vi "AlliGator Find FLI Dataset Paths.vi"(8 "error in (no error)":errorcluster, 11 "Path in":path) -> (0 "error out":errorcluster, 3 "Dataset Paths Array":path[](array[path]))   [LabVIEW 2021, in "AlliGator Files.lvlib"]
doc: "Analyze what type of files or folders the path contains."
uses:
  AlliGator Files.lvlib
  53ac5bec-de5c-4618-965b-4e0dad36e136.vi
  <vilib>/Utility/error.llb/Error Cluster From Error Code.vi
  <vilib>/ErrorRing/Error Ring.xnode
  <userlib>/_OpenG.lib/file/file.llb/openg_file.lvlib
panel:
  out "# Images":i32
  out "# Datasets":i32
  out "Gate Image Folder?":bool
  # "see the AlliGator License on the block diagram (Ctrl+E or Window:Show Block Diagram)"
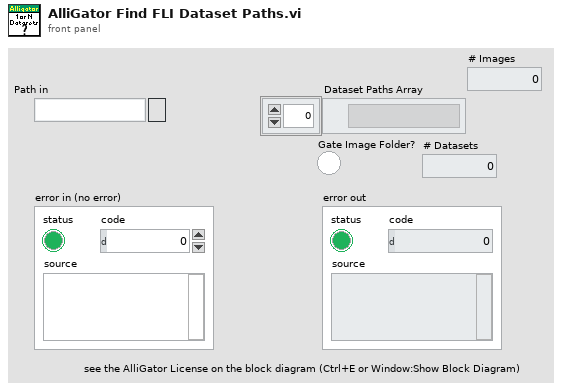
[diagram p1: front panel]
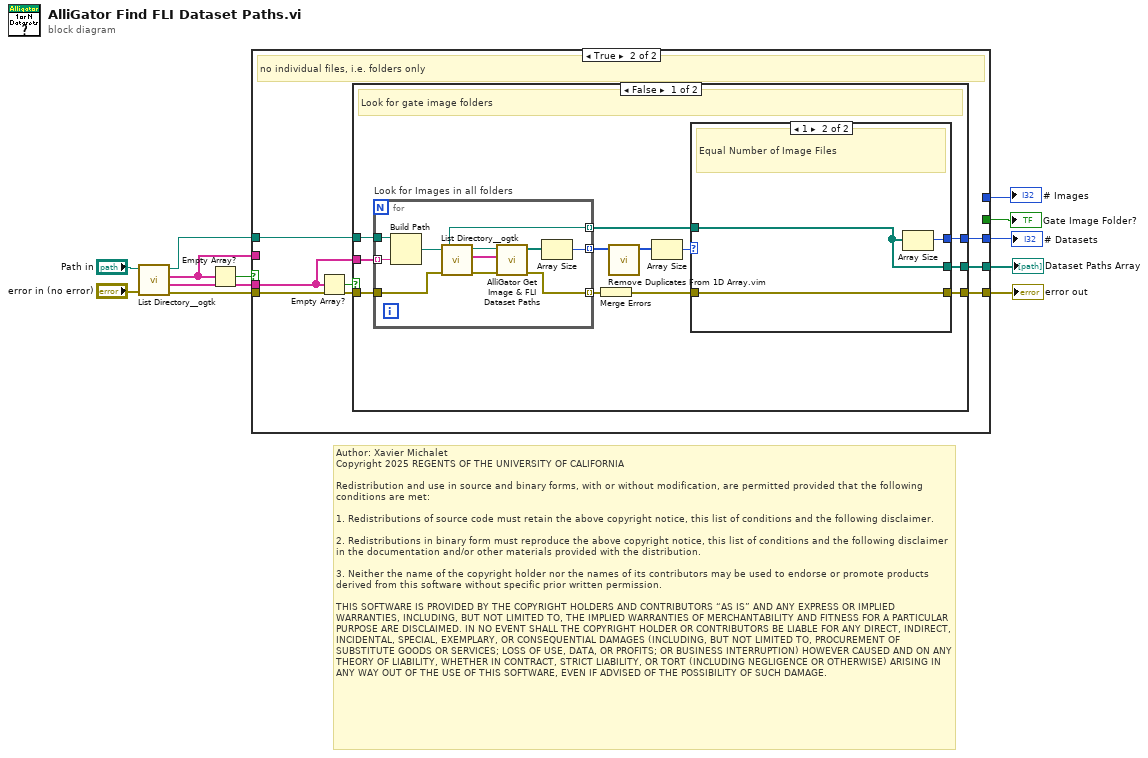
[diagram p0: block diagram]
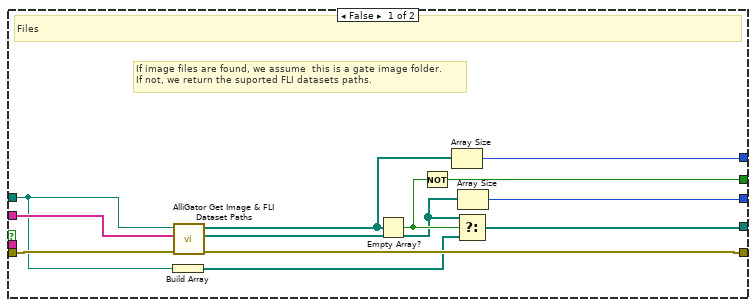
[diagram p2: hidden frame]
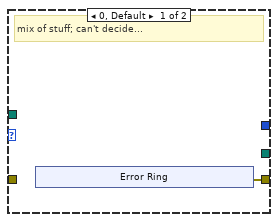
[diagram p3: hidden frame]
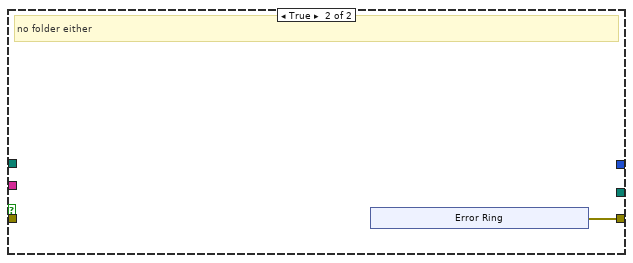
[diagram p4: hidden frame]
diagram:
  # "Author: Xavier Michalet\nCopyright 2025 REGENTS OF THE UNIVERSITY OF CALIFORNIA\n\nRedistribution and use in source and binary forms, with or without modification, are permitted provided that the following conditions are met:\n\n1. Redistributions of source code must retain the above copyright notice, this list of conditions and the following disclaimer.\n\n2. Redistributions in binary form must reproduce the above copyright notice, this list of conditions and the following disclaimer in the documentation and/or other materials provided with the distribution.\n\n3. Neither the name of the copyright holder nor the names of its contributors may be used to endorse or promote products derived from this software without specific prior written permission.\n\nTHIS SOFTWARE IS PROVIDED BY THE COPYRIGHT HOLDERS AND CONTRIBUTORS “AS IS” AND ANY EXPRESS OR IMPLIED WARRANTIES, INCLUDING, BUT NOT LIMITED TO, THE IMPLIED WARRANTIES OF MERCHANTABILITY AND FITNESS FOR A PARTICULAR PURPOSE ARE DISCLAIMED. IN NO EVENT SHALL THE COPYRIGHT HOLDER OR CONTRIBUTORS BE LIABLE FOR ANY DIRECT, INDIRECT, INCIDENTAL, SPECIAL, EXEMPLARY, OR CONSEQUENTIAL DAMAGES (INCLUDING, BUT NOT LIMITED TO, PROCUREMENT OF SUBSTITUTE GOODS OR SERVICES; LOSS OF USE, DATA, OR PROFITS; OR BUSINESS INTERRUPTION) HOWEVER CAUSED AND ON ANY THEORY OF LIABILITY, WHETHER IN CONTRACT, STRICT LIABILITY, OR TORT (INCLUDING NEGLIGENCE OR OTHERWISE) ARISING IN ANY WAY OUT OF THE USE OF THIS SOFTWARE, EVEN IF ADVISED OF THE POSSIBILITY OF SUCH DAMAGE."
  n1 = call <userlib>:"List Directory__ogtk.vi"("error in (no error)"="error in (no error)", "directory path"="Path in") -> ("error out"=w6:errorcluster, "directory names"=w4:string[], "file names"=w7:string[], "dup directory path"=w11:path)  [unwired: 2 in]
  n2 = Empty Array?(array=w7) -> (empty?=w8:bool)
  n3 = case shown="True" w8 {
    tunnel: [w22 w26] -> w12
    tunnel: w11 -> [w14 w28]
    tunnel: w7 -> [w24 _]
    tunnel: w6 -> [w23 w30]
    tunnel: [w21 w27] -> w5
    tunnel: w4 -> [_ w29]
    tunnel: [w19 _] -> w3
    tunnel: [w16 w25] -> w2
    tunnel: [w15 _] -> w1
    frame False {
      # "If image files are found, we assume  this is a gate image folder.\nIf not, we return the suported FLI datasets paths."
      # "Files"
      n4 = Build Array(w14) -> (w13:path[])
      n5 = call "AlliGator Get Image & FLI Dataset Paths.vi"("error in (no error)"=w23, "File names"=w24, "Directory path"=w14) -> ("error out"=w21:errorcluster, "FLI Dataset Paths"=w17:path[], "Image Paths"=w20:path[])  [unwired: 6 in]
      n6 = Empty Array?(array=w20) -> (empty?=w18:bool)
      n7 = Not(x=w18) -> (.not. x?=w19:bool)
      n8 = Array Size(array=w20) -> (size(s)=w15:i32)
      n9 = Select(t=w17, s=w18, f=w13) -> (s? t:f=w22:path[])
      n10 = Array Size(array=w17) -> (size(s)=w16:i32)
    }
    frame True {
      # "no individual files, i.e. folders only"
      n11 = Empty Array?(array=w29) -> (empty?=w31:bool)
      n12 = case shown="False" w31 {
        tunnel: w30 -> [w41 _]
        tunnel: [w34 w62] -> w27
        tunnel: w29 -> [w42 _]
        tunnel: w28 -> [w43 _]
        tunnel: [w37 _] -> w26
        tunnel: [w32 _] -> w25
        frame False {
          # "Look for gate image folders"
          n13 = for "Look for Images in all folders" {
            tunnel: w43 -> [w61]
            tunnel: w42 -> [w60] mode=indexing
            tunnel: w41 -> [w59]
            tunnel: [w55] -> w40 mode=indexing
            tunnel: [w53] -> w33 mode=indexing
            tunnel: [w52] -> w36 mode=indexing
            n14 = Build Path(base path=w61, name or relative path=w60) -> (appended path=w52:path)
            n15 = call <userlib>:"List Directory__ogtk.vi"("error in (no error)"=w59, "directory path"=w52) -> ("error out"=w56:errorcluster, "file names"=w57:string[], "dup directory path"=w58:path)  [unwired: 2 in, 1 out]
            n16 = call "AlliGator Get Image & FLI Dataset Paths.vi"("error in (no error)"=w56, "File names"=w57, "Directory path"=w58) -> ("error out"=w55:errorcluster, "Image Paths"=w54:path[])  [unwired: 6 in, 1 out]
            n17 = Array Size(array=w54) -> (size(s)=w53:i32)
          }
          n18 = Merge Errors(w40) -> (w35:errorcluster)
          n19 = call "Remove Duplicates From 1D Array.vim"("array"=w33) -> ("array with duplicates removed"=w39:i32[])  [unwired: 10 in]
          n20 = Array Size(array=w39) -> (size(s)=w38:i32)
          n21 = case shown="1" w38 {
            tunnel: [_ w50] -> w37
            tunnel: w36 -> [_ w50]
            tunnel: w35 -> [_ w51]
            tunnel: [w44 w51] -> w34
            tunnel: [_ w49] -> w32
            frame 0, Default {
              # "mix of stuff; can't decide..."
              n22 = xnode "Error Ring"() -> ("error out"=w44:errorcluster)
            }
            frame 1 {
              # "Equal Number of Image Files"
              n23 = Array Size(array=w50) -> (size(s)=w49:i32)
            }
          }
        }
        frame True {
          # "no folder either"
          n24 = xnode "Error Ring"() -> ("error out"=w62:errorcluster)
        }
      }
    }
  }
  "error out" <- w5
  "Dataset Paths Array" <- w12
  "Gate Image Folder?" <- w3
  "# Datasets" <- w2
  "# Images" <- w1
